vi "Autonomous Independent.vi"() -> ()   [LabVIEW 2018]
doc: "This VI is called when autonomous begins, and will automatically be terminated when autonomous ends. You can carry out timed or sensor driven robot movement independently without needing to return to the caller."
uses:
  <vilib>/Rock Robotics/WPI/ThirdParty/Phoenix-LabVIEW/Motor Controller/Controls/CTRE_Phoenix_MotorControl_ControlMode.ctl
  <vilib>/Rock Robotics/Network Tables/NT Read String.vi
  <vilib>/addons/control/pid/pid.llb/PID (DBL).vi
  <vilib>/Rock Robotics/WPI/ThirdParty/Phoenix-LabVIEW/Motor Controller/Get/CTRE_Phoenix_MotorController_GetSelectedSensorData.vi
  FIRST-3958-Controls-Library/NavX/navX Library v2/navX Library v2.lvlib
  <vilib>/addons/control/pid/NI_PID_pid.lvlib
panel:
  in  "10_strafe":dbl
  in  "angle_thresh":dbl
  in  "speed thresh":dbl
  in  "Angle PID":T1={"proportional gain (Kc)"=1.0, "integral time (Ti, min)"=0.01, "derivative time (Td, min)"=0.0} {"derivative time (Td, min)" format="%.3f"; "integral time (Ti, min)" format="%.3f"; "proportional gain (Kc)" format="%.3f"}
  in  "Array":cluster{"Action":string, "N1":dbl, "N2":dbl}[](array[cluster])=[{"Action"="Turn", "N1"=0.0, "N2"=0.6}, {"Action"="Turn", "N1"=0.0, "N2"=0.0}, {"Action"="Strafe", "N1"=0.0, "N2"=0.0}]
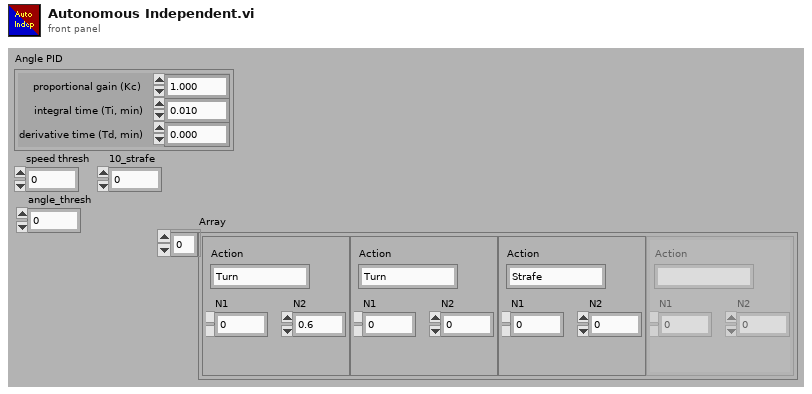
[diagram p1: front panel]
types:
  T1 = cluster{"proportional gain (Kc)":dbl, "integral time (Ti, min)":dbl, "derivative time (Td, min)":dbl}
  T2 = typedef "navX Library v2.lvlib/Z900_navX_DeviceTypeDef.ctl" = cluster{"Interface":cluster{"Protocol":T3, "Update Rate (4Hz-100Hz)":u8, "navX Open TypeDef":variant}, "Notify Packet":refnum<notifier>, "Loop VI Refnum":refnum<vi>, "Ready to Close Occurrence Refnum":refnum<k4>}
  T3 = typedef "navX Library v2.lvlib/Z900_navX_ProtocolTypeDef.ctl" = enum16{"SERIAL", "I2C", "SPI"}
  T4 = typedef "WPI_MotorControlDeviceRef.ctl" = cluster{"DeviceStatus":errorcluster, "Type":T5, "PWM":cluster{"PWM Channel":T6, "DeadBand":T7}, "CAN":cluster{"Device Number":u8, "SetOutput VI Ref":variant, "GetOutput VI Ref":variant, "Enable VI Ref":variant, "Disable VI Ref":variant, "Data":variant}, "Invert":bool, "DIO PWM":cluster{"PWM \"Enable\" Channel":T6, "DIOChannel":T8, "PWM Rate":dbl}}
  T5 = typedef "WPI_MotorControlType.ctl" = enum16{"PWM", "CAN", "DIO PWM"}
  T6 = typedef "FPGA_DIOPWMChannel.ctl" = enum8{"PWM 0", "PWM 1", "PWM 2", "PWM 3", "PWM 4", "PWM 5", "PWM 6", "PWM 7", "PWM 8", "PWM 9", "PWM MXP 0", "PWM MXP 1", "PWM MXP 2", "PWM MXP 3", "PWM MXP 4", "PWM MXP 5", "PWM MXP 6", "PWM MXP 7", "PWM MXP 8", "PWM MXP 9", "Invalid"}
  T7 = typedef "WPI_PWMDeadband.ctl" = cluster{"Name":string, "maxPositivePwm":i32, "minPositivePwm":i32, "centerPwm":i32, "maxNegativePwm":i32, "minNegativePwm":i32, "angularRange":u16}
  T8 = typedef "FPGA_DIOChannel.ctl" = enum8{"DIO 0", "DIO 1", "DIO 2", "DIO 3", "DIO 4", "DIO 5", "DIO 6", "DIO 7", "DIO 8", "DIO 9", "DIO MXP 0", "DIO MXP 1", "DIO MXP 2", "DIO MXP 3", "DIO MXP 4", "DIO MXP 5", "DIO MXP 6", "DIO MXP 7", "DIO MXP 8", "DIO MXP 9", "DIO MXP 10", "DIO MXP 11", "DIO MXP 12", "DIO MXP 13", "DIO MXP 14", "DIO MXP 15", "SPI Port CS1", "SPI Port CS2", "SPI Port CS3", "SPI Port MISO", "SPI Port MOSI", "Invalid"}
  T9 = typedef "CTRE_Phoenix_MotorControl_ControlMode.ctl" = u16
  T10 = cluster{"Yaw":dbl, "Roll":dbl, "Pitch":dbl, "Heading":dbl, "Fused Heading":dbl}
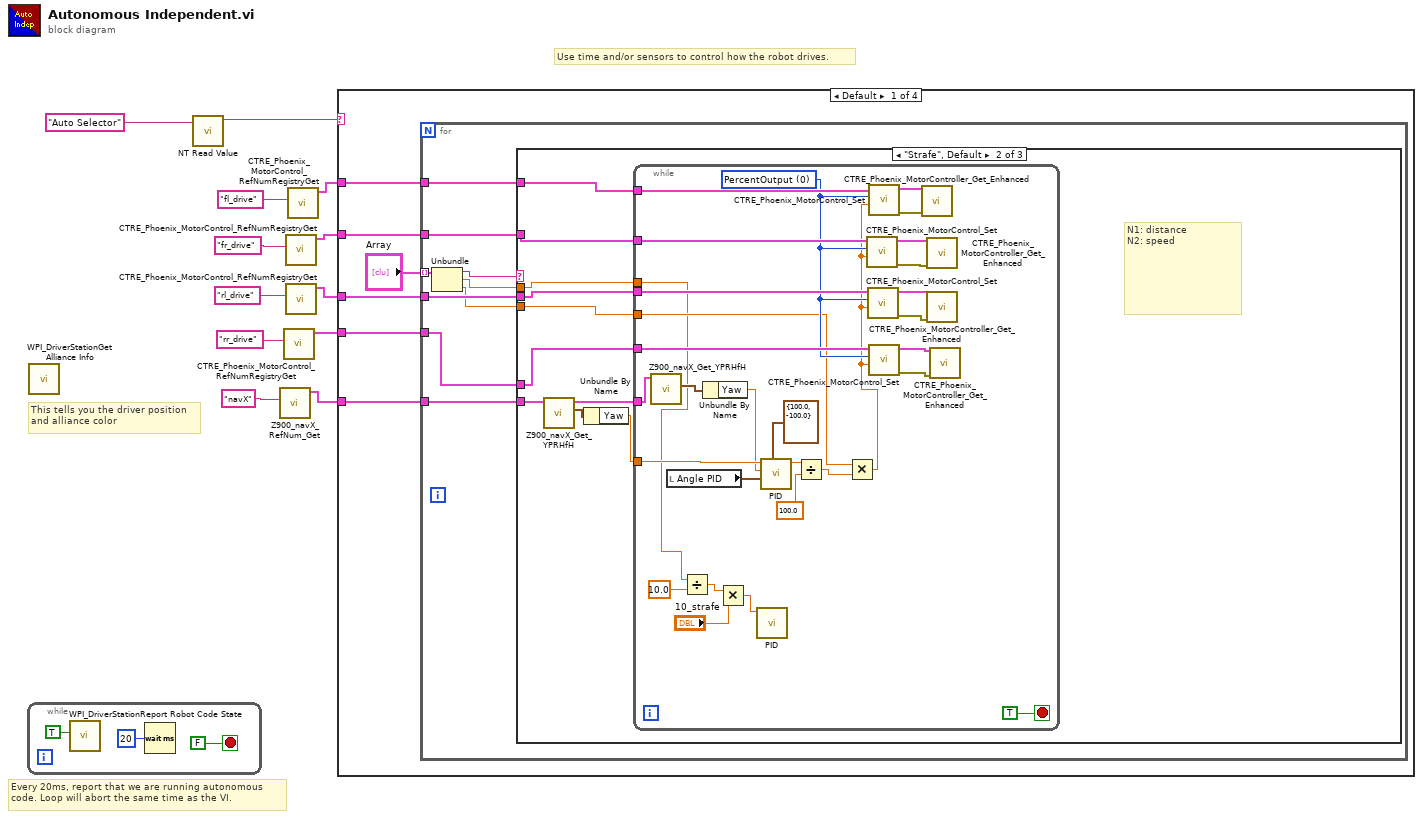
[diagram p0: block diagram]
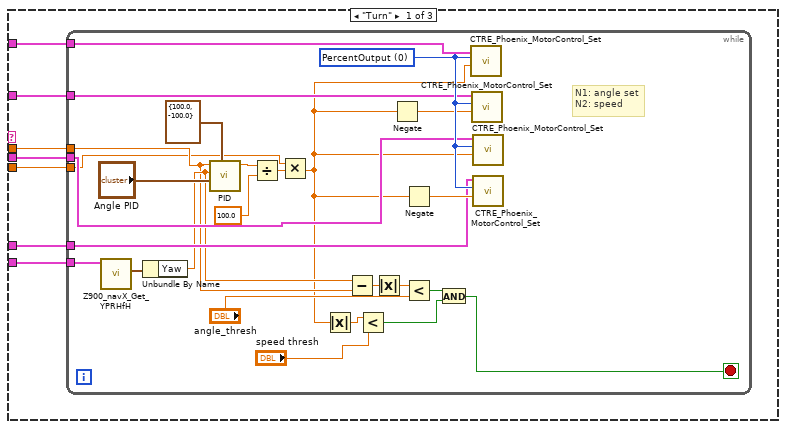
[diagram p2: hidden frame]
diagram:
  # "Every 20ms, report that we are running autonomous\ncode. Loop will abort the same time as the VI."
  # "Use time and/or sensors to control how the robot drives."
  # "This tells you the driver position\nand alliance color"
  n1 = while {
    stop <- FALSE stop-if-true
    n2 = call <vilib>:"WPI_DriverStationReport Robot Code State.vi"("Autonomous"=TRUE) -> ()  [unwired: 10 in, 1 out]
    n3 = Wait (ms)(milliseconds to wait=u32 20) -> ()  [unwired: 1 out]
  }
  n4 = call <vilib>:"WPI_DriverStationGet Alliance Info.vi"() -> ()  [unwired: 12 out]
  n5 = call-poly <vilib>:"NT Read Value.vi"("Name"="Auto Selector") -> ("String"=w11:string)  [unwired: 9 in, 1 out]
  n6 = call "Z900_navX_RefNum_Get.vi"("refnum name"="navX") -> ("navX Device"=w5:T2)  [unwired: 9 in, 1 out]
  n7 = call <vilib>:"CTRE_Phoenix_MotorControl_RefNumRegistryGet.vi"("refnum name"="rr_drive") -> ("PhoenixMotorControlDevRef"=w1:T4)  [unwired: 9 in, 1 out]
  n8 = call <vilib>:"CTRE_Phoenix_MotorControl_RefNumRegistryGet.vi"("refnum name"="fr_drive") -> ("PhoenixMotorControlDevRef"=w3:T4)  [unwired: 9 in, 1 out]
  n9 = call <vilib>:"CTRE_Phoenix_MotorControl_RefNumRegistryGet.vi"("refnum name"="rl_drive") -> ("PhoenixMotorControlDevRef"=w2:T4)  [unwired: 9 in, 1 out]
  n10 = call <vilib>:"CTRE_Phoenix_MotorControl_RefNumRegistryGet.vi"("refnum name"="fl_drive") -> ("PhoenixMotorControlDevRef"=w4:T4)  [unwired: 9 in, 1 out]
  n11 = case shown="Default" w11 {
    tunnel: w5 -> [w20 _ _ _]
    tunnel: w4 -> [w19 _ _ _]
    tunnel: w3 -> [w18 _ _ _]
    tunnel: w2 -> [w17 _ _ _]
    tunnel: w1 -> [w16 _ _ _]
    frame Default {
      n12 = for {
        tunnel: "Array" -> [w30] mode=indexing
        tunnel: w20 -> [w22]
        tunnel: w19 -> [w29]
        tunnel: w18 -> [w28]
        tunnel: w17 -> [w27]
        tunnel: w16 -> [w26]
        n13 = Unbundle(w30) -> ("Action"=w25:string, "N1"=w24:dbl, "N2"=w23:dbl)
        n14 = case shown="\"Strafe\", Default" w25 {
          tunnel: w22 -> [w37 w68 _]
          tunnel: w29 -> [w36 w73 _]
          tunnel: w28 -> [w35 w72 _]
          tunnel: w27 -> [w34 w71 _]
          tunnel: w26 -> [w33 w70 _]
          tunnel: w24 -> [w32 w64 _]
          tunnel: w23 -> [w31 w69 _]
          frame "Turn" {
            n15 = while {
              tunnel: w37 -> [w63]
              tunnel: w36 -> [w55]
              tunnel: w35 -> [w54]
              tunnel: w34 -> [w53]
              tunnel: w33 -> [w52]
              tunnel: w32 -> [w42]
              tunnel: w31 -> [w38]
              stop <- w45 stop-if-true
              w58 = T9 0 items=["PercentOutput"=0, "Position"=1, "Velocity"=2, "Current"=3, "Follower"=5, "MotionProfile"=6, "MotionMagic"=7, "MotionProfileArc"=10, "Disabled"=15] ("Control Mode")
              # "N1: angle set\nN2: speed"
              n16 = call "Z900_navX_Get_YPRHfH.vi"("navX Device"=w63) -> ("YRPHfH"=w62:T10)  [unwired: 7 in, 3 out]
              n17 = Unbundle By Name(w62) -> ("Yaw"=w51:dbl)
              n18 = call-poly <vilib>:"PID.vi"("output range"=cluster{"output high":dbl, "output low":dbl} {"output high"=100.0, "output low"=-100.0}, "PID gains"="Angle PID", "process variable"=w51, "setpoint"=w42) -> ("output"=w41:dbl)  [unwired: 6 in, 1 out]
              n19 = Divide(x=w41, y=100.0) -> (x/y=w39:dbl)
              n20 = Multiply(x=w38, y=w39) -> (x*y=w40:dbl)
              n21 = Absolute Value(x=w40) -> (abs(x)=w47:dbl)
              n22 = Subtract(x=w51, y=w42) -> (x-y=w50:dbl)
              n23 = Less?(x=w47, y="speed thresh") -> (x < y?=w46:bool)
              n24 = Absolute Value(x=w50) -> (abs(x)=w49:dbl)
              n25 = Negate(x=w40) -> (-x=w56:dbl)
              n26 = Negate(x=w40) -> (-x=w57:dbl)
              n27 = Less?(x=w49, y="angle_thresh") -> (x < y?=w48:bool)
              n28 = And(x=w48, y=w46) -> (x .and. y?=w45:bool)
              n29 = call <vilib>:"CTRE_Phoenix_MotorControl_Set.vi"("Output"=w40, "Control Mode"=w58, "PhoenixMotorControlDevRef"=w55) -> ()  [unwired: 7 in, 2 out]
              n30 = call <vilib>:"CTRE_Phoenix_MotorControl_Set.vi"("Output"=w56, "Control Mode"=w58, "PhoenixMotorControlDevRef"=w54) -> ()  [unwired: 7 in, 2 out]
              n31 = call <vilib>:"CTRE_Phoenix_MotorControl_Set.vi"("Output"=w40, "Control Mode"=w58, "PhoenixMotorControlDevRef"=w53) -> ()  [unwired: 7 in, 2 out]
              n32 = call <vilib>:"CTRE_Phoenix_MotorControl_Set.vi"("Output"=w57, "Control Mode"=w58, "PhoenixMotorControlDevRef"=w52) -> ()  [unwired: 7 in, 2 out]
            }
          }
          frame "Strafe", Default {
            # "N1: distance\nN2: speed"
            n33 = call "Z900_navX_Get_YPRHfH.vi"("navX Device"=w68) -> ("YRPHfH"=w67:T10, "navX Device"=w65:T2)  [unwired: 7 in, 2 out]
            n34 = Unbundle By Name(w67) -> ("Yaw"=w66:dbl)
            n35 = while {
              tunnel: w73 -> [w103]
              tunnel: w72 -> [w102]
              tunnel: w71 -> [w101]
              tunnel: w70 -> [w100]
              tunnel: w69 -> [w94]
              tunnel: w66 -> [w85]
              tunnel: w65 -> [w83]
              tunnel: w64 -> [w76]
              stop <- TRUE stop-if-true
              w99 = T9 0 items=["PercentOutput"=0, "Position"=1, "Velocity"=2, "Current"=3, "Follower"=5, "MotionProfile"=6, "MotionMagic"=7, "MotionProfileArc"=10, "Disabled"=15] ("Control Mode")
              n36 = call "Z900_navX_Get_YPRHfH.vi"("navX Device"=w83) -> ("YRPHfH"=w82:T10)  [unwired: 7 in, 3 out]
              n37 = local read "Angle PID"() -> (w84:T1)
              n38 = Divide(x=w76, y=10.0) -> (x/y=w79:dbl)
              n39 = Unbundle By Name(w82) -> ("Yaw"=w81:dbl)
              n40 = Multiply(x=w79, y="10_strafe") -> (x*y=w77:dbl)
              n41 = call-poly <vilib>:"PID.vi"("setpoint"=w77) -> ()  [unwired: 9 in, 2 out]
              n42 = call-poly <vilib>:"PID.vi"("output range"=cluster{"output high":dbl, "output low":dbl} {"output high"=100.0, "output low"=-100.0}, "PID gains"=w84, "process variable"=w81, "setpoint"=w85) -> ("output"=w98:dbl)  [unwired: 6 in, 1 out]
              n43 = Divide(x=w98, y=100.0) -> (x/y=w95:dbl)
              n44 = Multiply(x=w94, y=w95) -> (x*y=w75:dbl)
              n45 = call <vilib>:"CTRE_Phoenix_MotorControl_Set.vi"("Output"=w75, "Control Mode"=w99, "PhoenixMotorControlDevRef"=w102) -> ("error out"=w90:errorcluster, "PhoenixMotorControlDevRef"=w91:T4)  [unwired: 7 in]
              n46 = call <vilib>:"CTRE_Phoenix_MotorControl_Set.vi"("Output"=w75, "Control Mode"=w99, "PhoenixMotorControlDevRef"=w101) -> ("error out"=w88:errorcluster, "PhoenixMotorControlDevRef"=w89:T4)  [unwired: 7 in]
              n47 = call <vilib>:"CTRE_Phoenix_MotorControl_Set.vi"("Output"=w75, "Control Mode"=w99, "PhoenixMotorControlDevRef"=w103) -> ("error out"=w92:errorcluster, "PhoenixMotorControlDevRef"=w93:T4)  [unwired: 7 in]
              n48 = call <vilib>:"CTRE_Phoenix_MotorControl_Set.vi"("Output"=w75, "Control Mode"=w99, "PhoenixMotorControlDevRef"=w100) -> ("error out"=w86:errorcluster, "PhoenixMotorControlDevRef"=w87:T4)  [unwired: 7 in]
              n49 = call-poly <vilib>:"CTRE_Phoenix_MotorController_Get_Enhanced.vi"("PhoenixMotorControlDevRef"=w93, "error in"=w92) -> ()  [unwired: 10 in, 4 out]
              n50 = call-poly <vilib>:"CTRE_Phoenix_MotorController_Get_Enhanced.vi"("PhoenixMotorControlDevRef"=w91, "error in"=w90) -> ()  [unwired: 10 in, 4 out]
              n51 = call-poly <vilib>:"CTRE_Phoenix_MotorController_Get_Enhanced.vi"("PhoenixMotorControlDevRef"=w89, "error in"=w88) -> ()  [unwired: 10 in, 4 out]
              n52 = call-poly <vilib>:"CTRE_Phoenix_MotorController_Get_Enhanced.vi"("PhoenixMotorControlDevRef"=w87, "error in"=w86) -> ()  [unwired: 10 in, 4 out]
            }
          }
          frame "Forward" {
            # "N1: distance\nN2: speed"
          }
        }
      }
    }
    frame "Alternative 1" {
    }
    frame "Alternative 2" {
    }
    frame "Your Turn" {
    }
  }
